vi "GetSelectedItemName_RCM.vi"(0 "Display State In":T1={"RCM File Path"=path "", "Left"=300, "Top"=300, "Font Name"="Tahoma", "Font Size"=13, "Font Color"=0, "Separator Color"=9868950, "Frame Color"=9868950, "Overlay Color"=26367}, 9 "Container State":T2, 11 "error in (no error)":errorcluster) -> (4 "Display State Out":T1={"RCM File Path"=path "", "Left"=300, "Top"=300, "Font Name"="Tahoma", "Font Size"=13, "Font Color"=0, "Separator Color"=9868950, "Frame Color"=9868950, "Overlay Color"=26367}, 6 "Item Name":string, 8 "Selected?":bool, 15 "error out":errorcluster)   [LabVIEW 2009, in "RCM.xctl"]
uses:
  RCM.xctl
  <vilib>/_xctls/Container State.ctl
  Ability/State_RCM.ctl
  <vilib>/_xctls/XControlSupport.lvlib
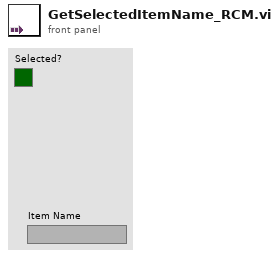
[diagram p1: front panel]
types:
  T1 = typedef "RCM.xctl/State_RCM.ctl" = cluster{"RCM File Path":path, "Left":u32, "Top":u32, "Font Name":string, "Font Size":i16, "Font Color":u32, "Separator Color":u32, "Frame Color":u32, "Overlay Color":u32}
  T2 = typedef "XControlSupport.lvlib/Container State.ctl" = cluster{"Indicator?":bool, "Run Mode?":bool, " Refnum":refnum<vi>}
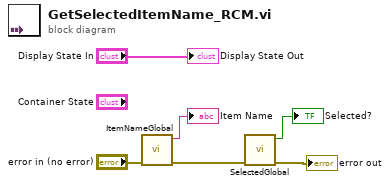
[diagram p0: block diagram]
diagram:
  n1 = call "ItemNameGlobal.vi"("error in (no error)"="error in (no error)") -> ("error out"=w3:errorcluster, "item name out"=→"Item Name":string)  [unwired: 9 in]
  n2 = call "SelectedGlobal.vi"("error in (no error)"=w3) -> ("error out"=→"error out":errorcluster, "selected out out"=→"Selected?":bool)  [unwired: 9 in]
  "Display State Out" <- "Display State In"
